vi "Configure Glitch Trigger Source.vi"(0 "VISA Resource Name":refnum<visa-resource-name>, 1 "Glitch Polarity (Positive)":i32(slide), 5 "Trigger Source (Channel 1)":string(combo)="CHAN1", 7 "Trigger Level (0.0 V)":dbl format="%^.2e", 9 "Glitch Width (30.0E-9 s)":dbl=3e-08 format="%^.2e", 11 "error in (no error)":errorcluster {"code" format="%.0x"}, 12 "Glitch Condition (Less Than)":string(combo)="LESS") -> (4 "VISA Resource Name Out":refnum<visa-resource-name>, 15 "error out":errorcluster {"code" format="%.0x"})   [LabVIEW 2011, in "Agilent 546XX Series.lvlib"]
doc: "This VI configures the glitch trigger. A glitch trigger occurs when the trigger signal has a pulse with a width that is less than the glitch width when the glitch trigger condition is set to less than, or a pulse with a width that is greater than the glitch width when the glitch trigger condition is set to greater than, or a pulse with a width that is less than the upper glitch width range value and greater than the lower glitch width range value when the glitch trigger condition is set to in range. You specify the glitch width in the Glitch Width control. You specify the upper glitch width range value and lower glitch width range value using the VI ag546xx Configure Glitch Trigger Range. You specify the polarity of the pulse with the Glitch Polarity control. The trigger does not actually occur until the edge of a pulse that corresponds to the Glitch Width and Glitch Polarity crosses the threshold you specify in the Trigger Level control. \n\nNotes:\n\n(1) This VI affects instrument behavior only if the Trigger Type is Glitch Trigger. Call the ag546xx Configure Trigger VI to set the Trigger Type before you call this VI."
uses:
  Agilent 546XX Series.lvlib
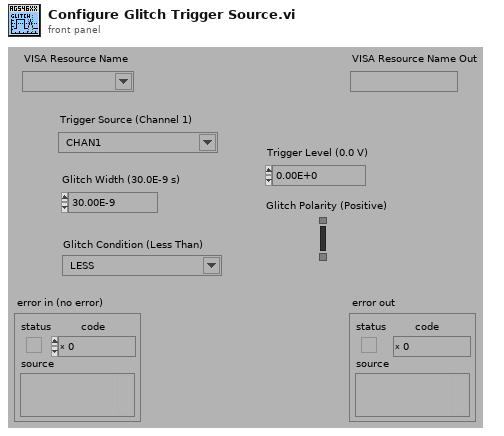
[diagram p1: front panel]
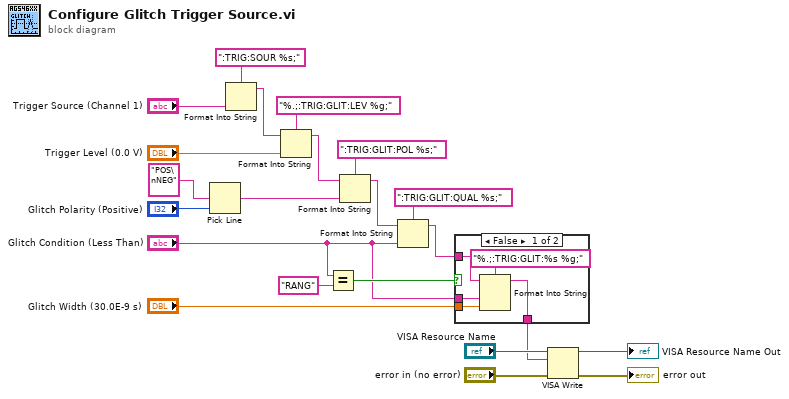
[diagram p0: block diagram]
diagram:
  n1 = Pick Line(multi-line string="POS\nNEG", line index="Glitch Polarity (Positive)") -> (output string=w5:string)  [unwired: 1 in]
  n2 = Format Into String(format string=":TRIG:SOUR %s;", "Trigger Source (Channel 1)") -> (resulting string=w7:string)  [unwired: 2 in, 1 out]
  n3 = Format Into String(format string="%.;:TRIG:GLIT:LEV %g;", initial string=w7, "Trigger Level (0.0 V)") -> (resulting string=w8:string)  [unwired: 1 in, 1 out]
  n4 = Equal?(x="Glitch Condition (Less Than)", y="RANG") -> (x = y?=w2:bool)
  n5 = Format Into String(format string=":TRIG:GLIT:POL %s;", initial string=w8, w5) -> (resulting string=w9:string)  [unwired: 1 in, 1 out]
  n6 = Format Into String(format string=":TRIG:GLIT:QUAL %s;", initial string=w9, "Glitch Condition (Less Than)") -> (resulting string=w10:string)  [unwired: 1 in, 1 out]
  n7 = case shown="False" w2 {
    tunnel: w10 -> [w26 w28]
    tunnel: [w25 w28] -> w6
    tunnel: "Glitch Width (30.0E-9 s)" -> [w24 _]
    tunnel: "Glitch Condition (Less Than)" -> [w23 _]
    frame False {
      n8 = Format Into String(format string="%.;:TRIG:GLIT:%s %g;", initial string=w26, w23, w24) -> (resulting string=w25:string)  [unwired: 1 in, 1 out]
    }
    frame True {
    }
  }
  n9 = VISA Write(VISA resource name="VISA Resource Name", write buffer=w6, error in (no error)="error in (no error)") -> (VISA resource name out=→"VISA Resource Name Out":refnum<visa-resource-name>, error out=→"error out":errorcluster)  [unwired: 1 out]
